vi "Test Command To Wash State.vi"(8 "error in (no error)":errorcluster, 11 "TestCase in":refnum<class "CarWashTestCases.lvclass">) -> (0 "error out":errorcluster, 3 "TestCase out":refnum<class "CarWashTestCases.lvclass">)   [LabVIEW 2018, in "CarWashTestCases.lvclass"]
uses:
  CarWashTestCases.lvclass
  Command.ctl
  Position.ctl
  <vilib>/addons/_JKI Toolkits/VI Tester/TestCase.llb/TestCase.lvclass
  C:/Program Files (x86)/National Instruments/LabVIEW 2018/vi.lib/addons/_JKI Toolkits/VI Tester/TestCase.llb/TestCase.lvclass
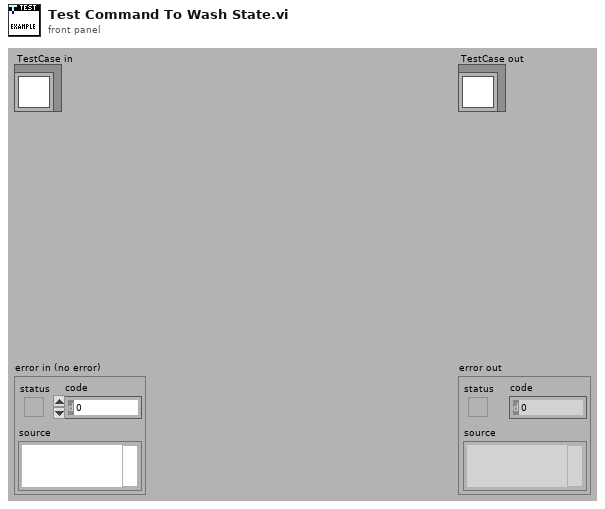
[diagram p1: front panel]
types:
  T1 = typedef "Position.ctl" = enum32{"Under Body Wash Position", "Main Wash Position", "Air Dry Position"}
  T2 = typedef "Command.ctl" = enum16{"Underbody Wash", "Soap Application", "Main High-Pressure Wash", "Clear Water Rinse", "Air Dry Cycle", "Stop"}
  T3 = typedef "MessageQueueData.ctl" = cluster{"State":T2, "Data":variant}
  T4 = typedef "WashState.ctl" = cluster{"Time Remaining":i32, "LastTickCount":i32, "Required Vehicle Position":T1}
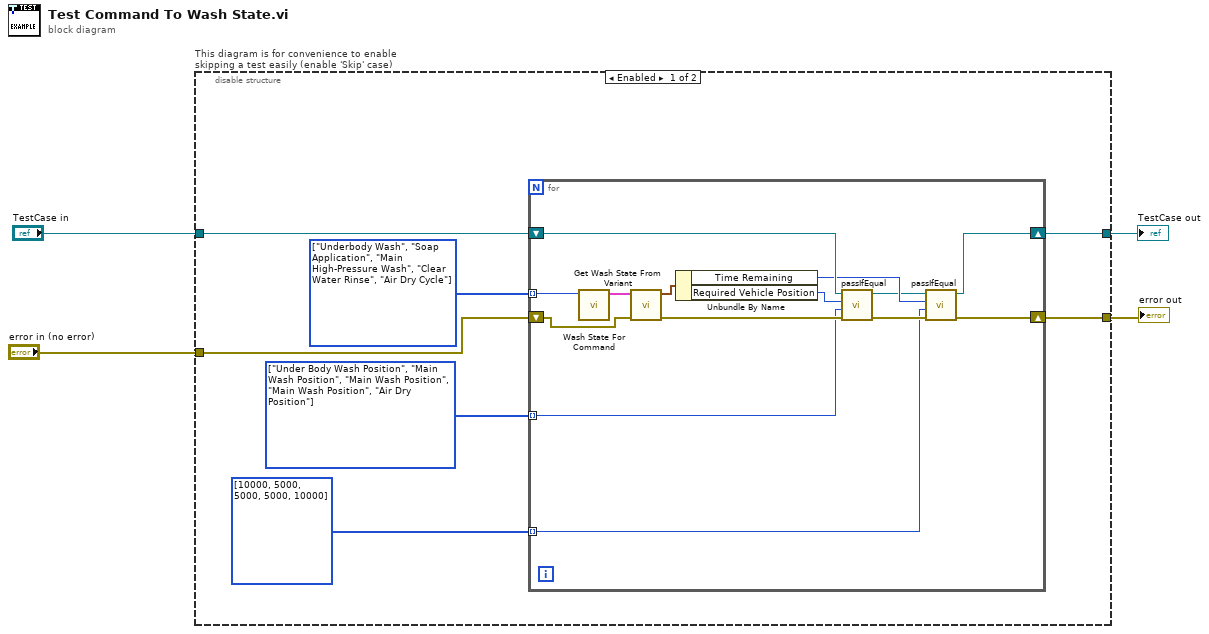
[diagram p0: block diagram]
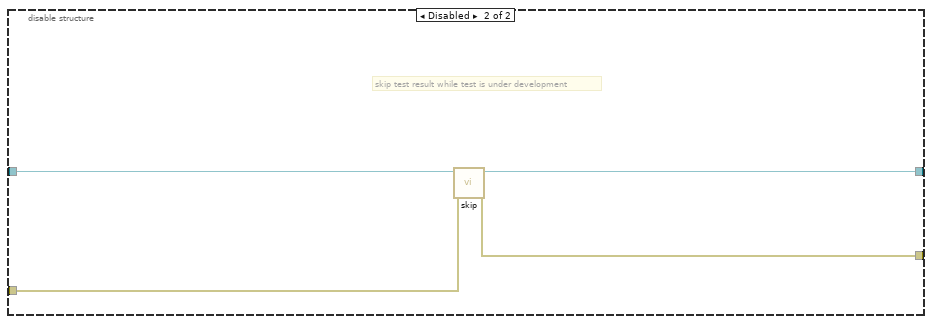
[diagram p2: hidden frame]
diagram:
  n1 = disable-structure "This diagram is for convenience to enable skipping a test easily (enable 'Skip' case)" shown="Enabled" {
    disable-tunnel: "TestCase in" -> [w9 w29]
    disable-tunnel: [w6 w27] -> w1
    disable-tunnel: [w5 w28] -> w3
    disable-tunnel: "error in (no error)" -> [w10 w26]
    frame Enabled {
      w8 = T1[] [enum."Under Body Wash Position", enum."Main Wash Position", enum."Main Wash Position", enum."Main Wash Position", enum."Air Dry Position"] items=["Under Body Wash Position", "Main Wash Position", "Air Dry Position"]
      w11 = T2[] [enum."Underbody Wash", enum."Soap Application", enum."Main High-Pressure Wash", enum."Clear Water Rinse", enum."Air Dry Cycle"] items=["Underbody Wash", "Soap Application", "Main High-Pressure Wash", "Clear Water Rinse", "Air Dry Cycle", "Stop"]
      n2 = for {
        tunnel: w11 -> [w25] mode=indexing
        shift-right: [w13] -> w5
        shift-left: w10 -> [w23]
        tunnel: w8 -> [w15] mode=indexing
        tunnel: i32[] [10000, 5000, 5000, 5000, 10000] -> [w14] mode=indexing
        shift-right: [w12] -> w6
        shift-left: w9 -> [w19]
        n3 = call "Wash State For Command.vi"("Command"=w25) -> ("Queue Data for Command"=w24:T3)  [unwired: 10 in]
        n4 = call "Get Wash State From Variant.vi"("error in"=w23, "Message Queue Data"=w24) -> ("error out"=w22:errorcluster, "WashState out"=w21:T4)  [unwired: 8 in]
        n5 = Unbundle By Name(w21) -> ("Time Remaining"=w17:i32, "Required Vehicle Position"=w20:T1)
        n6 = call-dynamic "passIfEqual.vi"("error in (no error)"=w22, "y"=w15, "x"=w20, "TestCase in"=w19) -> ("error out"=w18:errorcluster, "TestCase out"=w16:refnum<class "CarWashTestCases.lvclass">)  [unwired: 6 in]
        n7 = call-dynamic "passIfEqual.vi"("error in (no error)"=w18, "y"=w14, "x"=w17, "TestCase in"=w16) -> ("error out"=w13:errorcluster, "TestCase out"=w12:refnum<class "CarWashTestCases.lvclass">)  [unwired: 6 in]
      }
    }
    frame Disabled {
      # "skip test result while test is under development"
      n8 = call <vilib>:"skip.vi"("error in (no error)"=w26, "TestCase in"=w29) -> ("error out"=w28:errorcluster, "TestCase out"=w27:refnum<class "CarWashTestCases.lvclass">)  [unwired: 8 in]
    }
  }
  "error out" <- w3
  "TestCase out" <- w1
